vi "GlobalGetMesaurementStatus.vi"() -> ()   [LabVIEW 2011]
panel:
  out "MeasurementAktiv":bool
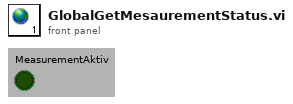
[diagram p1: front panel]
diagram:
